vi "12- Data entry with Cluster.vi"() -> ()   [LabVIEW 2019]
panel:
  in  "?":bool
  out "Phone":string
  out "Address":string
  out "Name":string
  in  "Cluster":T1
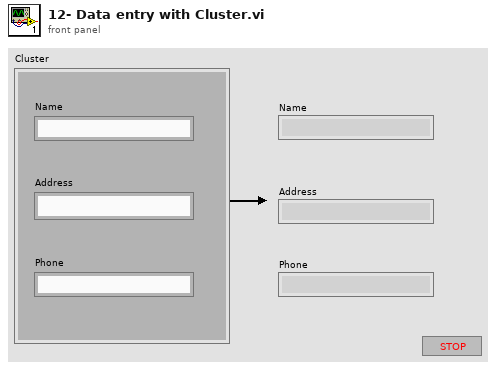
[diagram p1: front panel]
types:
  T1 = cluster{"Name":string, "Address":string, "Phone":string}
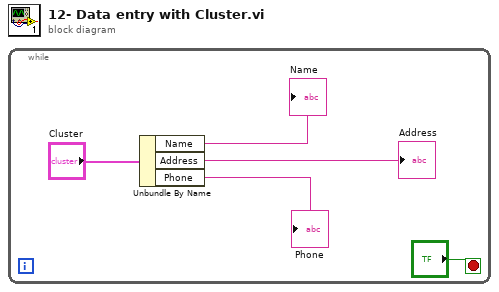
[diagram p0: block diagram]
diagram:
  n1 = while {
    stop <- "?" stop-if-true
    n2 = Unbundle By Name("Cluster") -> ("Name"=→"Name":string, "Address"=→"Address":string, "Phone"=→"Phone":string)
  }
